vi "Contour Line_Check Connected Contour Points.vi"(10 "edge 2":T1, 11 "edge 1":T1) -> (1 "connected?":bool, 2 "edge 2 out":T1, 3 "edge 1 out":T1)   [LabVIEW 2017, in "NI_AAL_Geometry.lvlib"]
uses:
  <vilib>/Analysis/NI_AAL_Geometry.lvlib
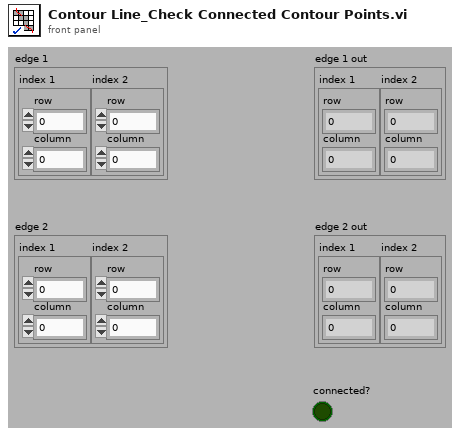
[diagram p1: front panel]
types:
  T1 = cluster{"index 1":cluster{"row":i32, "column":i32}, "index 2":cluster{"row":i32, "column":i32}}
  T2 = cluster{"index 1":cluster{"row":i32, "column":i32}, "index 2":cluster{"row":i32, "column":i32}}[]
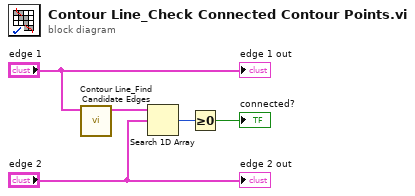
[diagram p0: block diagram]
diagram:
  n1 = call <vilib>:"Contour Line_Find Candidate Edges.vi"("edge"="edge 1") -> ("Candidate Edges"=w4:T2)  [unwired: 10 out]
  n2 = Search 1D Array(1D array=w4, element="edge 2") -> (index of element=w2:i32)  [unwired: 1 out]
  n3 = Greater Or Equal To 0?(x=w2) -> (x >= 0?=→"connected?":bool)
  "edge 1 out" <- "edge 1"
  "edge 2 out" <- "edge 2"
